vi "Create Folder.vi"(8 "error in":errorcluster, 11 "Path in":path) -> (0 "error out":errorcluster, 3 "Path out":path)   [LabVIEW 2019]
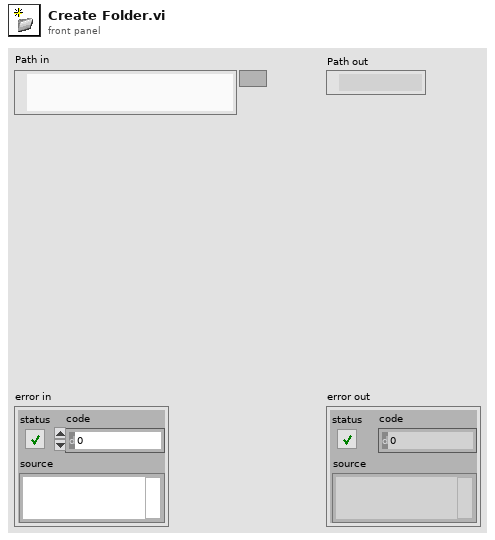
[diagram p1: front panel]
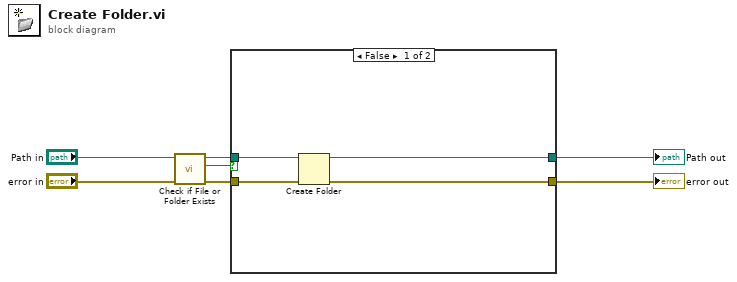
[diagram p0: block diagram]
diagram:
  n1 = call <vilib>:"Check if File or Folder Exists.vi"("error in (no error)"="error in", "path"="Path in") -> ("error out"=w5:errorcluster, "file or folder exists?"=w4:bool, "dup path"=w3:path)  [unwired: 7 in]
  n2 = case shown="False" w4 {
    tunnel: w5 -> [w11 w13]
    tunnel: w3 -> [w10 w12]
    tunnel: [w9 w13] -> w2
    tunnel: [w8 w12] -> w1
    frame False {
      n3 = Create Folder(path (use dialog)=w10, error in=w11) -> (created path=w8:path, error out=w9:errorcluster)  [unwired: 1 in, 1 out]
    }
    frame True {
    }
  }
  "error out" <- w2
  "Path out" <- w1
